vi "Test Make.vi"() -> ()   [LabVIEW 2019]
panel:
  in  "Btn Copy":bool
  in  "Copy To Folder":path=path "C:/Users/CHIAM KOK THIAM/Downloads/tdk/check double click/tdms/2 bumps"
  in  "Move To Folder":path=path "C:/Users/CHIAM KOK THIAM/Downloads/tdk/check double click/tdms/2 bumps"
  out "Last File":path
  in  "Btn Move":bool
  in  "Btn Stop":bool
  in  "Result":i32(listbox)
  in  "file path (dialog if empty)":path=path "C:/Users/CHIAM KOK THIAM/Downloads/tdk/check double click/tdms/1 bump"
  out "Peak Indexes":i32[](array[numeric])
  out "Waveform Graph 2":dbl[](graph)
  out "Waveform Graph":waveform(dbl)(graph)
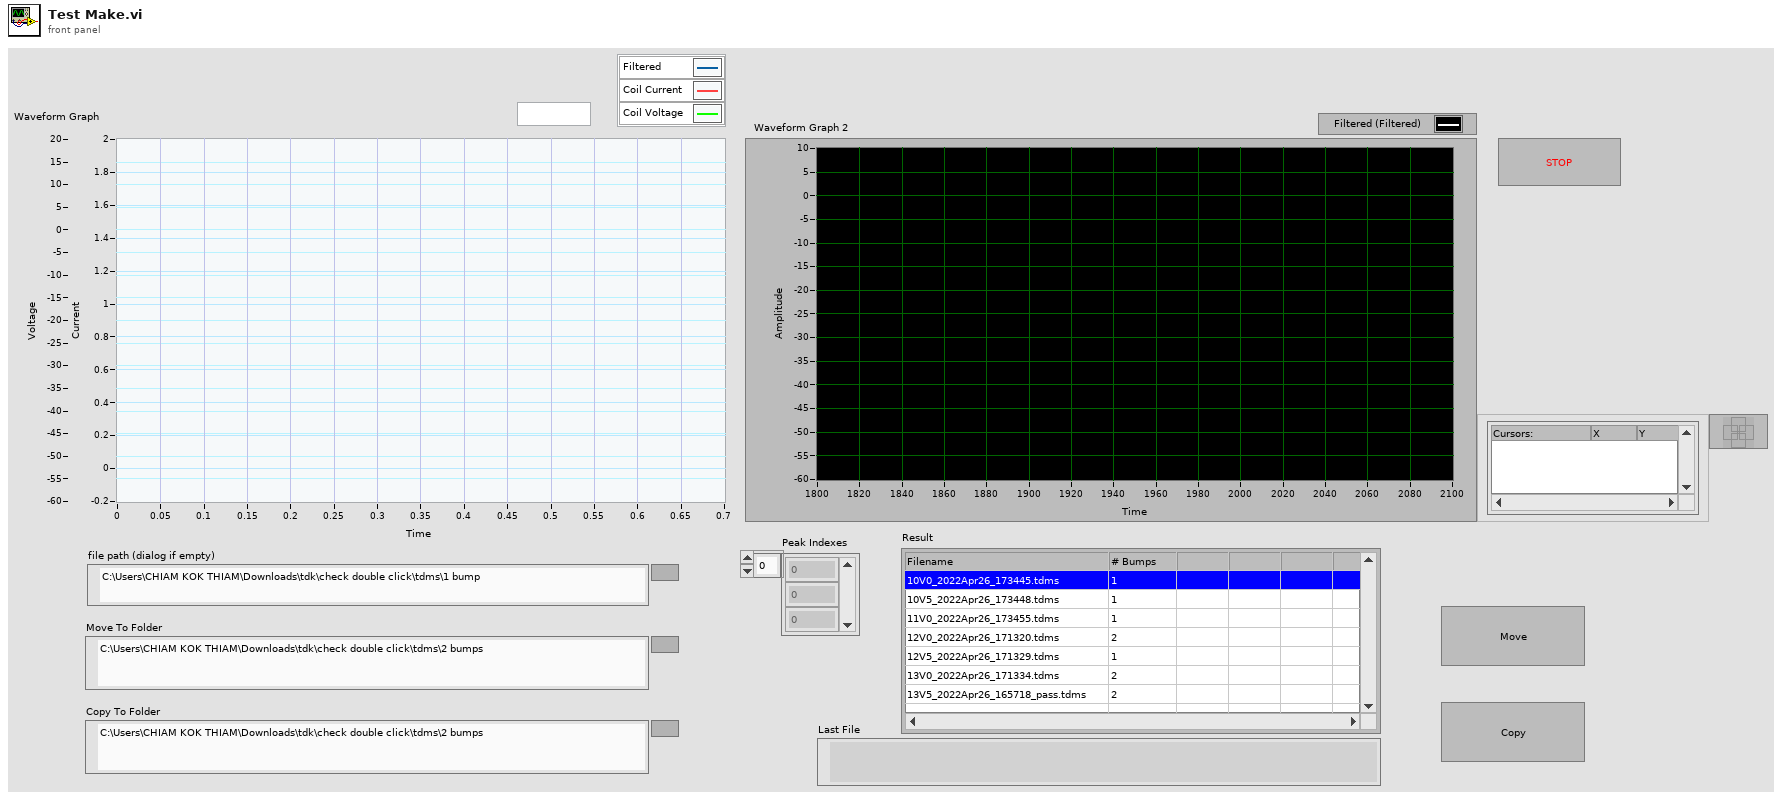
[diagram p1: front panel]
types:
  T1 = cluster{"Name":string, "Color":u32, "Style":u8, "Point Style":u8, "Name Visible":bool, "Allow Drag":bool, "Cursor Mode":u32, "Plot":i32, "Index":i32, "Position":cluster{"X":dbl, "Y":dbl}, "X Scale":u32, "Y Scale":u32, "Watch Plots":i32[], "Watch All Plots":bool, "Plot Area":i32, "Label Offset":cluster{"X":dbl, "Y":dbl}}
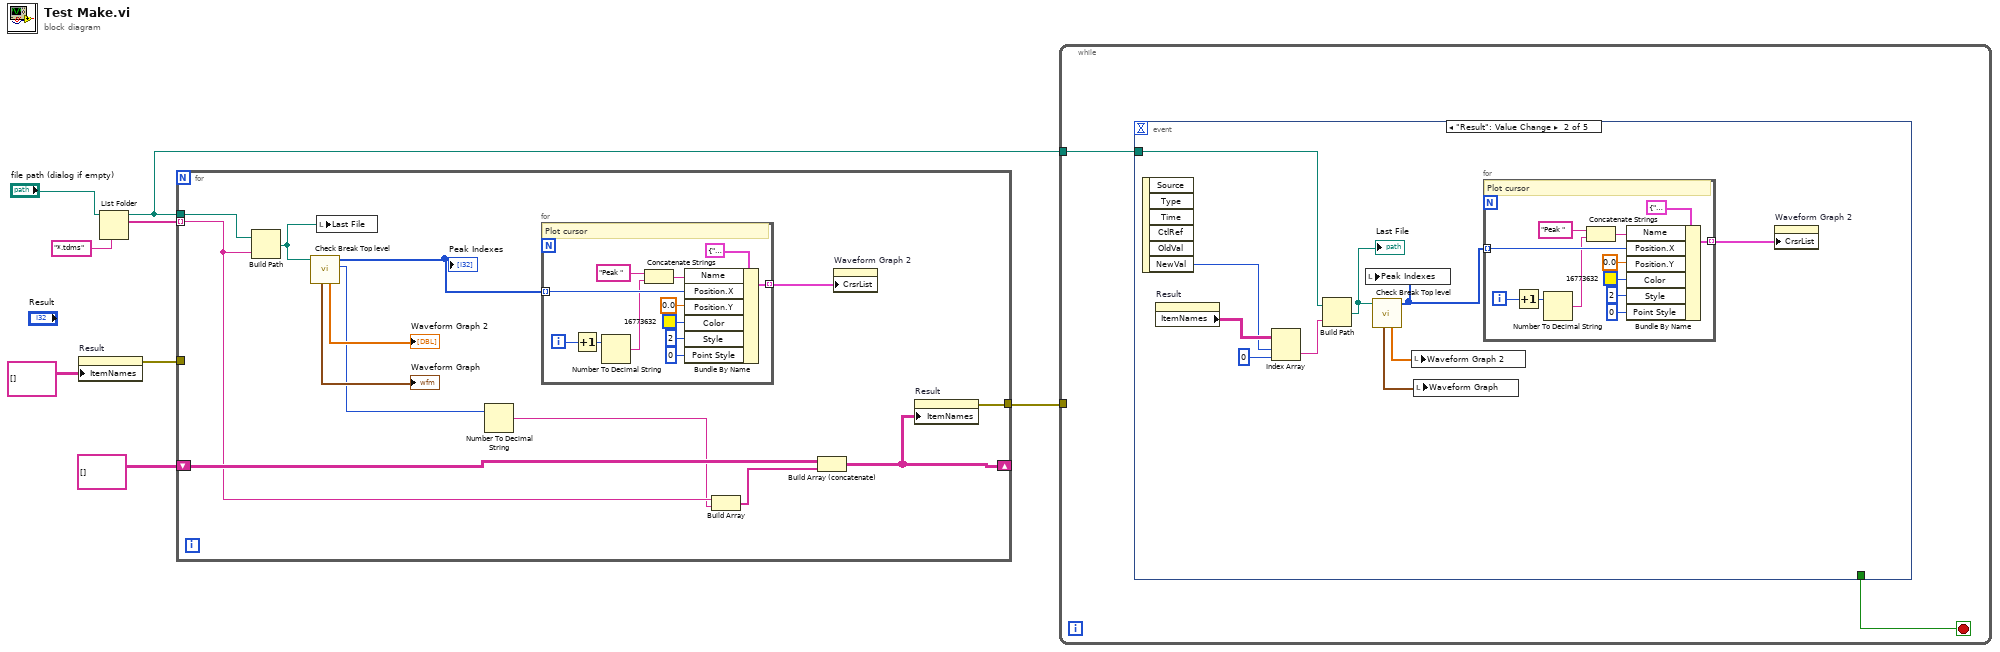
[diagram p0: block diagram]
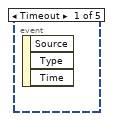
[diagram p2: hidden frame]
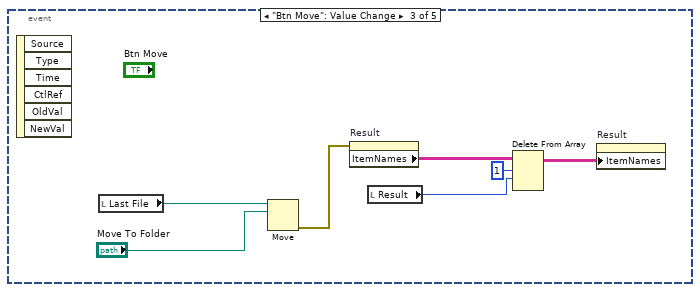
[diagram p3: hidden frame]
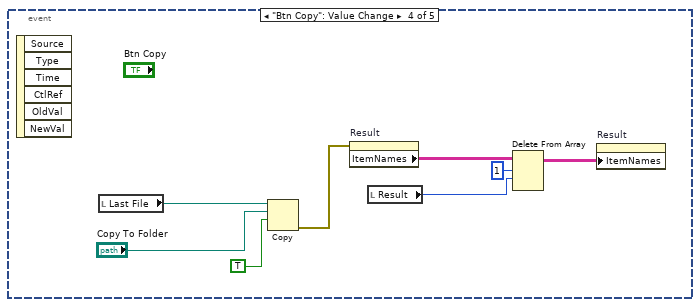
[diagram p4: hidden frame]
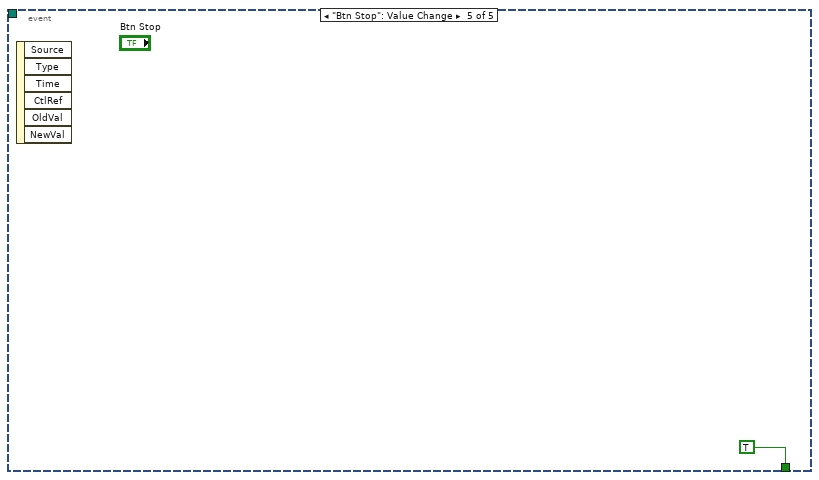
[diagram p5: hidden frame]
diagram:
  n1 = property on="Result" class="MCListbox (strict)"("ItemNames"=string[][] [] ("Item Names")) -> (error out=w3:errorcluster)  [unwired: 2 in, 1 out]
  n2 = List Folder(path="file path (dialog if empty)", pattern="*.tdms") -> (path out=w1:path, filenames=w7:string[])  [unwired: 2 in, 2 out]
  n3 = for {
    tunnel: w7 -> [w14] mode=indexing
    tunnel: w1 -> [w17]
    shift-right: [w11] -> _
    shift-left: string[][] [] -> [w15]
    tunnel: w3 -> [_]
    tunnel: [w10] -> w2
    n4 = Build Path(base path=w17, name or relative path=w14) -> (appended path=w9:path)
    n5 = call "Check Break Top level.vi"("path"=w9) -> ("Number of Peaks"=w16:i32, "Peak Indexes"=w20:i32[], "Y"=→"Waveform Graph 2":dbl[], "Waveform Graph"=→"Waveform Graph":waveform(dbl))  [unwired: 6 in, 1 out]
    "Peak Indexes" <- w20
    n6 = local write "Last File"(w9) -> ()
    n7 = Number To Decimal String(number=w16) -> (decimal integer string=w13:string)  [unwired: 1 in]
    n8 = for {
      tunnel: w20 -> [w30] mode=indexing
      tunnel: [w31] -> w19 mode=indexing
      i -> [w33]
      # "Plot cursor"
      n9 = Increment(x=w33) -> (x+1=w32:i32)
      n10 = Number To Decimal String(number=w32) -> (decimal integer string=w27:string)  [unwired: 1 in]
      n11 = Concatenate Strings("Peak " ("Name"), w27) -> (w29:string)
      n12 = Bundle By Name(cluster=T1 {"Name"="", "Color"=0, "Style"=0, "Point Style"=0, "Name Visible"=FALSE, "Allow Drag"=FALSE, "Cursor Mode"=0, "Plot"=0, "Index"=0, "Position"={"X"=0.0, "Y"=0.0}, "X Scale"=0, "Y Scale"=0, "Watch Plots"=[], "Watch All Plots"=FALSE, "Plot Area"=0, "Label Offset"={"X"=0.0, "Y"=0.0}}, "Name"=w29, "Position.X"=w30, "Position.Y"=0.0 ("Position.X"), "Color"=u32 16773632, "Style"=u8 2, "Point Style"=u8 0) -> (w31:T1)
    }
    n13 = Build Array(w14, w13) -> (w12:string[])
    n14 = Build Array (concatenate)(w15, w12) -> (w11:string[][])
    n15 = property on="Waveform Graph 2" class="WFGraph (strict)"("CrsrList"=w19) -> ()  [unwired: 2 in, 2 out]
    n16 = property on="Result" class="MCListbox (strict)"("ItemNames"=w11) -> (error out=w10:errorcluster)  [unwired: 2 in, 1 out]
  }
  n17 = while {
    tunnel: w2 -> [_]
    tunnel: w1 -> [w35]
    stop <- w34 stop-if-true
    n18 = event shown="[1] \"Result\": Value Change" {
      selector: _ -> [_ _ _ _ _]
      dyn-events: _ -> [_ _ _ _ _]
      timeout: _ -> [_ _ _ _ _]
      tunnel: w35 -> [_ w41 _ _ _]
      tunnel: [_ _ _ _ TRUE] -> w34
      event Timeout {
        n19 = event-data() -> ()  [unwired: 1 in, 3 out]
      }
      event "Result": Value Change {
        n20 = event-data() -> ("NewVal"=w44:i32)  [unwired: 1 in, 5 out]
        n21 = property on="Result" class="MCListbox (strict)"() -> ("ItemNames"=w45:string[][])  [unwired: 2 in, 2 out]
        n22 = Index Array(array=w45, index (row)=w44, index (col)=0 ("disabled index (col)")) -> (element=w42:string)
        n23 = Build Path(base path=w41, name or relative path=w42) -> (appended path=w40:path)
        "Last File" <- w40
        n24 = call "Check Break Top level.vi"("path"=w40) -> ("Peak Indexes"=w36:i32[], "Y"=w39:dbl[], "Waveform Graph"=w38:waveform(dbl))  [unwired: 6 in, 2 out]
        n25 = local write "Peak Indexes"(w36) -> ()
        n26 = local write "Waveform Graph 2"(w39) -> ()
        n27 = local write "Waveform Graph"(w38) -> ()
        n28 = for {
          tunnel: w36 -> [w54] mode=indexing
          tunnel: [w55] -> w37 mode=indexing
          i -> [w57]
          # "Plot cursor"
          n29 = Increment(x=w57) -> (x+1=w56:i32)
          n30 = Number To Decimal String(number=w56) -> (decimal integer string=w51:string)  [unwired: 1 in]
          n31 = Concatenate Strings("Peak " ("Name"), w51) -> (w53:string)
          n32 = Bundle By Name(cluster=T1 {"Name"="", "Color"=0, "Style"=0, "Point Style"=0, "Name Visible"=FALSE, "Allow Drag"=FALSE, "Cursor Mode"=0, "Plot"=0, "Index"=0, "Position"={"X"=0.0, "Y"=0.0}, "X Scale"=0, "Y Scale"=0, "Watch Plots"=[], "Watch All Plots"=FALSE, "Plot Area"=0, "Label Offset"={"X"=0.0, "Y"=0.0}}, "Name"=w53, "Position.X"=w54, "Position.Y"=0.0 ("Position.X"), "Color"=u32 16773632, "Style"=u8 2, "Point Style"=u8 0) -> (w55:T1)
        }
        n33 = property on="Waveform Graph 2" class="WFGraph (strict)"("CrsrList"=w37) -> ()  [unwired: 2 in, 2 out]
      }
      event "Btn Move": Value Change {
        n34 = event-data() -> ()  [unwired: 1 in, 6 out]
        n35 = local read "Last File"() -> (w64:path)
        n36 = Move(source path=w64, 10:"Move To Folder") -> (error out=w58:errorcluster)  [unwired: 3 in, 2 out]
        n37 = property on="Result" class="MCListbox (strict)"(error in=w58) -> ("ItemNames"=w62:string[][])  [unwired: 1 in, 2 out]
        n38 = local read "Result"() -> (w60:i32)
        n39 = Delete From Array(array=w62, length=1, index (row)=w60) -> (array with subset deleted=w61:string[][])  [unwired: 1 in, 1 out]
        n40 = property on="Result" class="MCListbox (strict)"("ItemNames"=w61) -> ()  [unwired: 2 in, 2 out]
      }
      event "Btn Copy": Value Change {
        n41 = event-data() -> ()  [unwired: 1 in, 6 out]
        n42 = local read "Last File"() -> (w72:path)
        n43 = Copy(9:TRUE ("overwrite (F)"), 10:"Copy To Folder", 11:w72) -> (0:w66:errorcluster)  [unwired: 2 in, 2 out]
        n44 = property on="Result" class="MCListbox (strict)"(error in=w66) -> ("ItemNames"=w70:string[][])  [unwired: 1 in, 2 out]
        n45 = local read "Result"() -> (w68:i32)
        n46 = Delete From Array(array=w70, length=1, index (row)=w68) -> (array with subset deleted=w69:string[][])  [unwired: 1 in, 1 out]
        n47 = property on="Result" class="MCListbox (strict)"("ItemNames"=w69) -> ()  [unwired: 2 in, 2 out]
      }
      event "Btn Stop": Value Change {
        n48 = event-data() -> ()  [unwired: 1 in, 6 out]
      }
    }
  }
